vi "Remove Oldest Duplicates.vi"(8 "error in":errorcluster, 11 "XML Document in":refnum<class "XML Document.lvclass">) -> (0 "error out":errorcluster, 3 "XML Document out":refnum<class "XML Document.lvclass">)   [LabVIEW 2014, in "XML Document.lvclass"]
uses:
  XML Document.lvclass
  Node_class/Node.lvclass
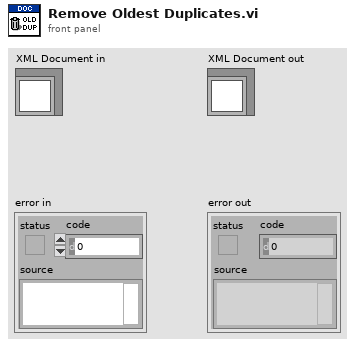
[diagram p1: front panel]
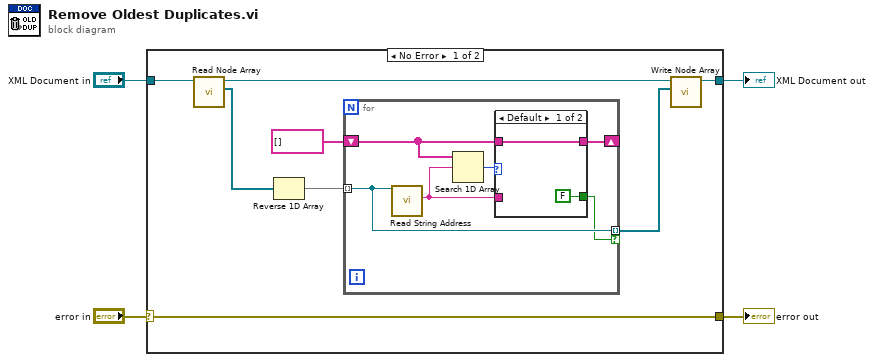
[diagram p0: block diagram]
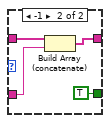
[diagram p2: hidden frame]
diagram:
  n1 = case shown="No Error" "error in" {
    selector: "error in" -> [w11 w26]
    tunnel: [w11 w26] -> w3
    tunnel: [w6 w25] -> w1
    tunnel: "XML Document in" -> [w12 w25]
    frame No Error {
      n2 = call-dynamic "Read Node Array.vi"("XML Document in"=w12) -> ("Node Array"=w9:refnum<class "Node.lvclass">[], "XML Document out"=w10:refnum<class "XML Document.lvclass">)  [unwired: 8 in, 1 out]
      n3 = Reverse 1D Array(array=w9) -> (reversed array=w7:refnum<class "Node.lvclass">[])
      n4 = for {
        tunnel: w7 -> [w14] mode=indexing
        shift-right: [w16] -> _
        shift-left: string[] [] -> [w17]
        tunnel: [w14] -> w5 mode=indexing if=w13
        n5 = call-dynamic "Read String Address.vi"("Node in"=w14) -> ("String Address"=w15:string)  [unwired: 8 in, 2 out]
        n6 = Search 1D Array(1D array=w17, element=w15) -> (index of element=w18:i32)  [unwired: 1 in]
        n7 = case shown="Default" w18 {
          tunnel: w17 -> [w20 w24]
          tunnel: [w20 w22] -> w16
          tunnel: w15 -> [_ w23]
          tunnel: [FALSE TRUE] -> w13
          frame Default {
          }
          frame -1 {
            n8 = Build Array (concatenate)(w24, w23) -> (w22:string[])
          }
        }
      }
      n9 = call-dynamic "Write Node Array.vi"("Node Array"=w5, "XML Document in"=w10) -> ("XML Document out"=w6:refnum<class "XML Document.lvclass">)  [unwired: 8 in, 1 out]
    }
    frame Error {
    }
  }
  "error out" <- w3
  "XML Document out" <- w1
